vi "Cleanup.vi"(10 "Critical Stop?":bool, 11 "Panel Actor in":refnum<class "Panel Actor.lvclass">) -> ()   [LabVIEW 2017, in "MGI-Panel Actor.lvlib" / "Panel Actor.lvclass"]
doc: "Throws the \"Stopped\" event and destroys all references.\n----\nCopyright: MGI 2018\nAuthor: Derek Trepanier"
uses:
  Panel Actor.lvclass
  Panel Actor.lvclass/Panel Actor.ctl
  panel-manager/Source/Panel/Panel.lvclass
  panel-manager/Source/Panel Helper/Panel Helper.lvclass
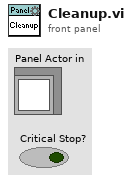
[diagram p1: front panel]
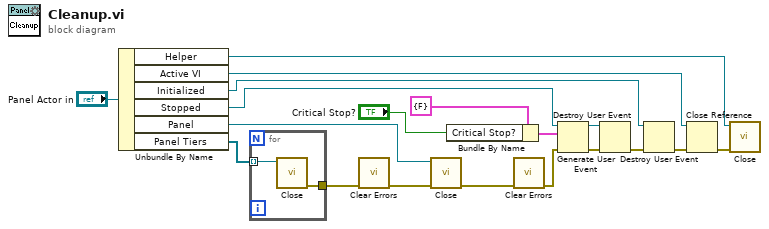
[diagram p0: block diagram]
diagram:
  n1 = Unbundle By Name("Panel Actor in") -> ("Helper"=w18:refnum<class "Panel Helper.lvclass">, "Active VI"=w17:refnum<vi>, "Initialized"=w3:refnum<user-event>, "Stopped"=w11:refnum<user-event>, "Panel"=w10:refnum<class "Panel.lvclass">, "Panel Tiers"=w8:refnum<class "Panel.lvclass">[])
  n2 = for {
    tunnel: w8 -> [w21] mode=indexing
    tunnel: [w20] -> w7
    n3 = call-dynamic "Close.vi"("Panel In"=w21) -> ("Error Out"=w20:errorcluster)  [unwired: 10 in]
  }
  n4 = call <vilib>:"Clear Errors.vi"("error in (no error)"=w7) -> ("error out"=w6:errorcluster)  [unwired: 5 in, 1 out]
  n5 = call-dynamic "Close.vi"("Error In"=w6, "Panel In"=w10) -> ("Error Out"=w15:errorcluster)  [unwired: 9 in]
  n6 = Bundle By Name(cluster=cluster{"Critical Stop?":bool} {"Critical Stop?"=FALSE} ("event data"), "Critical Stop?"="Critical Stop?") -> (w13:cluster{"Critical Stop?":bool})
  n7 = call <vilib>:"Clear Errors.vi"("error in (no error)"=w15) -> ("error out"=w16:errorcluster)  [unwired: 5 in, 1 out]
  n8 = Generate User Event(user event=w11, event data cluster=w13, error in=w16) -> (user event out=w5:refnum<user-event>, error out=w4:errorcluster)  [unwired: 1 in]
  n9 = Destroy User Event(user event=w5, error in=w4) -> (error out=w2:errorcluster)
  n10 = Destroy User Event(user event=w3, error in=w2) -> (error out=w1:errorcluster)
  n11 = Close Reference(reference=w17, error in (no error)=w1) -> (error out=w19:errorcluster)
  n12 = call "Close.vi"("error in (no error)"=w19, "Controller in"=w18) -> ()  [unwired: 9 in, 1 out]
